vi "Consolidate Plot Configuration Information.vi"(9 "Plot Channel Configurations":T1[](array[typedef]), 10 "Variable Descriptions":T2[](array[typedef]), 11 "Variable References":refnum<k21>[](array[refnum])) -> (1 "Plot Channel Configurations":T1[](array[typedef]))   [LabVIEW 2017, in "DTacq Plot Display Library.lvlib"]
uses:
  DTacq Plot Display Library.lvlib
  Network Shared Variables/Typedefs/Shared Variable Properties--Cluster.ctl
  Typedefs/Plot Channel Configruation--Cluster.ctl
  Network Shared Variables/Shared Variables Library.lvlib
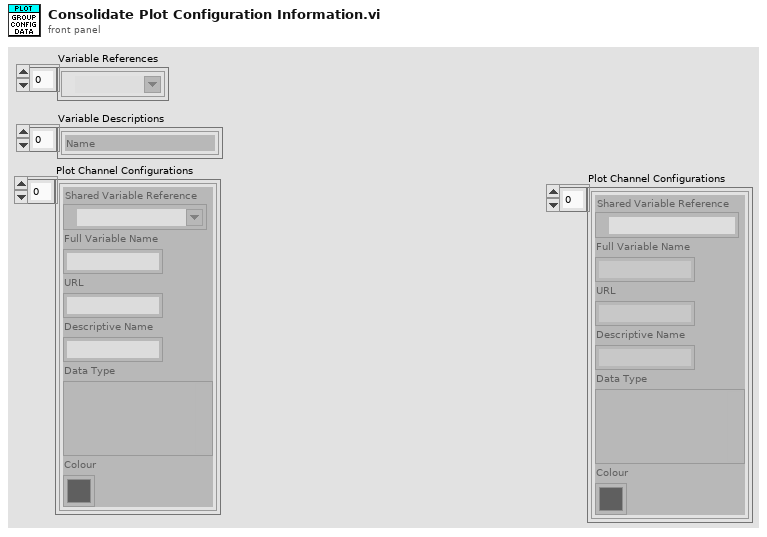
[diagram p1: front panel]
types:
  T1 = typedef "DTacq Plot Display Library.lvlib/Plot Channel Configruation--Cluster.ctl" = cluster{"Shared Variable Reference":refnum<k21>, "Full Variable Name":string, "URL":string, "Descriptive Name":string, "Data Type":variant, "Colour":u32}
  T2 = typedef "Shared Variables Library.lvlib/Shared Variable Properties--Cluster.ctl" = cluster{"Name":string, "URL":string, "Data Type":variant}
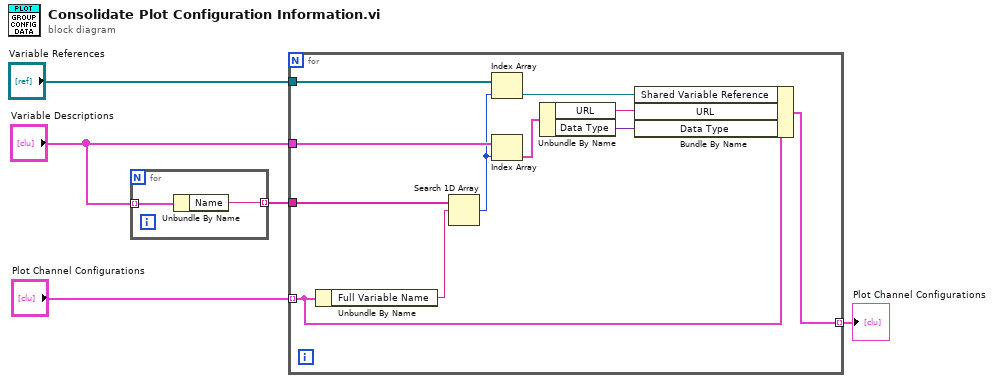
[diagram p0: block diagram]
diagram:
  n1 = for {
    tunnel: "Variable Descriptions" -> [w7] mode=indexing
    tunnel: [w6] -> w2 mode=indexing
    n2 = Unbundle By Name(w7) -> ("Name"=w6:string)
  }
  n3 = for {
    tunnel: "Plot Channel Configurations" -> [w16] mode=indexing
    tunnel: "Variable References" -> [w15]
    tunnel: "Variable Descriptions" -> [w13]
    tunnel: w2 -> [w18]
    tunnel: [w8] -> w1 mode=indexing
    n4 = Unbundle By Name(w16) -> ("Full Variable Name"=w17:string)
    n5 = Search 1D Array(1D array=w18, element=w17) -> (index of element=w12:i32)  [unwired: 1 in]
    n6 = Index Array(array=w15, index=w12) -> (element=w14:refnum<k21>)
    n7 = Index Array(array=w13, index=w12) -> (element=w11:T2)
    n8 = Unbundle By Name(w11) -> ("URL"=w10:string, "Data Type"=w9:variant)
    n9 = Bundle By Name(cluster=w16, "Shared Variable Reference"=w14, "URL"=w10, "Data Type"=w9) -> (w8:T1)
  }
  "Plot Channel Configurations" <- w1
